vi "ND to 1D.vi"(1 "ND Array":dbl[][](array[numeric])) -> (0 "1D Array":dbl[](array[numeric]))   [LabVIEW 2020]
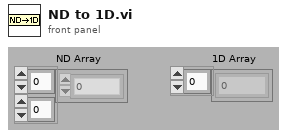
[diagram p1: front panel]
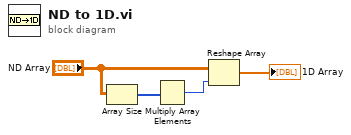
[diagram p0: block diagram]
diagram:
  n1 = Array Size(array="ND Array") -> (size(s)=w4:i32[])
  n2 = Multiply Array Elements(1:w4) -> (0:w1:i32)
  n3 = Reshape Array("ND Array", w1) -> (→"1D Array":dbl[])
